vi "InitializeProjectWizardItem.vi"(8 "error in (no error)":errorcluster, 9 "wizard argument":string, 10 "wizard":string, 11 "ProjectWizard in":refnum<class "ProjectWizard.lvclass">) -> (0 "error out":errorcluster, 3 "ProjectWizard out":refnum<class "ProjectWizard.lvclass">)   [LabVIEW 2009, in "NavScreen.lvlib" / "ProjectWizard.lvclass"]
uses:
  ProjectWizard.lvclass
  ProjectWizard.lvclass/ProjectWizard.ctl
  NavScreen.lvlib
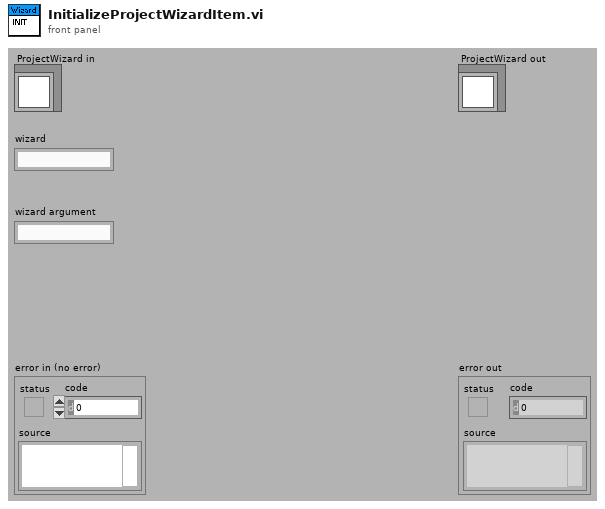
[diagram p1: front panel]
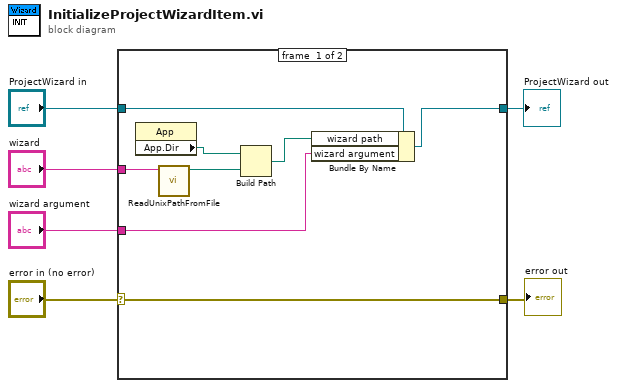
[diagram p0: block diagram]
diagram:
  n1 = case shown="No Error" "error in (no error)" {
    selector: "error in (no error)" -> [w14 w16]
    tunnel: [w14 w16] -> w5
    tunnel: [w12 w15] -> w3
    tunnel: "ProjectWizard in" -> [w13 w15]
    tunnel: "wizard argument" -> [w11 _]
    tunnel: "wizard" -> [w10 _]
    frame #0 {
      n2 = property class="App"() -> ("App.Dir"=w9:path)  [unwired: 2 in, 2 out]
      n3 = call "ReadUnixPathFromFile.vi"("path"=w10) -> ("path"=w8:path)  [unwired: 10 in]
      n4 = Build Path(base path=w9, name or relative path=w8) -> (appended path=w7:path)
      n5 = Bundle By Name(cluster=w13, "wizard path"=w7, "wizard argument"=w11) -> (w12:refnum<class "ProjectWizard.lvclass">)
    }
    frame #1 {
    }
  }
  "error out" <- w5
  "ProjectWizard out" <- w3
